vi "Camera-Events2Case.vi"(2 "OldVal":T2 {"Camera Parameters"."Pixel Format" items=["PIXEL_FORMAT_MONO8", "PIXEL_FORMAT_MONO16", "PIXEL_FORMAT_YUV422", "PIXEL_FORMAT_BAYER8_GRBG", "PIXEL_FORMAT_BAYER16_GRBG", "PIXEL_FORMAT_RGB24", "PIXEL_FORMAT_RGB48", "PIXEL_FORMAT_BAYER8_RGGB", "PIXEL_FORMAT_BAYER8_GBRG ", "PIXEL_FORMAT_BAYER8_BGGR ", "PIXEL_FORMAT_BAYER16_RGGB ", "PIXEL_FORMAT_BAYER16_GBRG", "PIXEL_FORMAT_BAYER16_BGGR", "PIXEL_FORMAT_RGB32"]}, 3 "NewVal":T2 {"Camera Parameters"."Pixel Format" items=["PIXEL_FORMAT_MONO8", "PIXEL_FORMAT_MONO16", "PIXEL_FORMAT_YUV422", "PIXEL_FORMAT_BAYER8_GRBG", "PIXEL_FORMAT_BAYER16_GRBG", "PIXEL_FORMAT_RGB24", "PIXEL_FORMAT_RGB48", "PIXEL_FORMAT_BAYER8_RGGB", "PIXEL_FORMAT_BAYER8_GBRG ", "PIXEL_FORMAT_BAYER8_BGGR ", "PIXEL_FORMAT_BAYER16_RGGB ", "PIXEL_FORMAT_BAYER16_GBRG", "PIXEL_FORMAT_BAYER16_BGGR", "PIXEL_FORMAT_RGB32"]}) -> (0 "Cameara Cambio Array":T3(array[ring]), 1 "Camara Cambio?":bool)   [LabVIEW 2010]
uses:
  <vilib>/addons/PixeLINK/Low Level Functions/CAMERA_FEATURES.llb/TDPU-CameraFeatures-PixelFormat.ctl
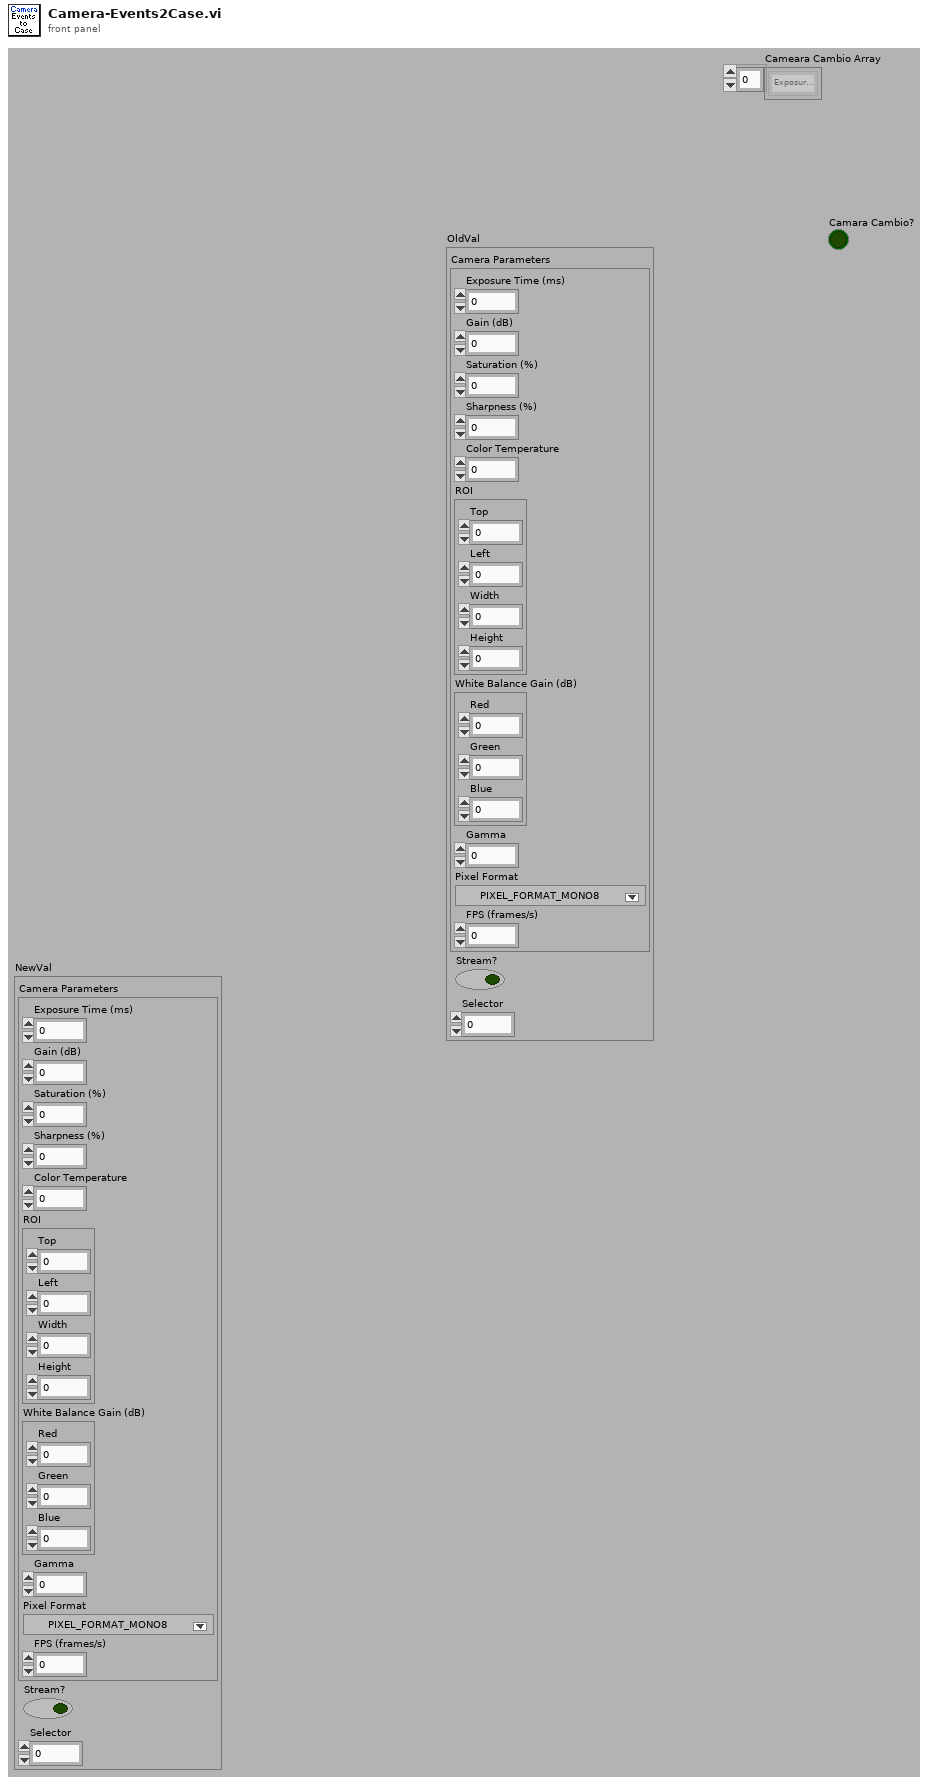
[diagram p1: front panel]
types:
  T1 = typedef "TDPU-CameraFeatures-PixelFormat.ctl" = u16
  T2 = cluster{"Camera Parameters":cluster{"Exposure Time (ms)":dbl, "Gain (dB)":dbl, "Saturation (%)":dbl, "Sharpness (%)":dbl, "Color Temperature":dbl, "ROI":cluster{"Top":i32, "Left":i32, "Width":i32, "Height":i32}, "White Balance Gain (dB)":cluster{"Red":dbl, "Green":dbl, "Blue":dbl}, "Gamma":dbl, "Pixel Format":T1, "FPS (frames/s)":i32}, "Stream?":bool, "Selector":u16}
  T3 = enum16{"Exposure Time (ms)", "Gain (dB)", "Saturation (%)", "Sharpness (%)", "Color Temperature (%)", "ROI", "White Balance Gain (dB)", "Gamma", "Pixel Format", "FPS (frames/s)", "Selector", "Stream", "Nothing"}[]
  T4 = cluster{"Top":i32, "Left":i32, "Width":i32, "Height":i32}
  T5 = enum16{"Exposure Time (ms)", "Gain (dB)", "Saturation (%)", "Sharpness (%)", "Color Temperature (%)", "ROI", "White Balance Gain (dB)", "Gamma", "Pixel Format", "FPS (frames/s)", "Selector", "Stream", "Nothing"}
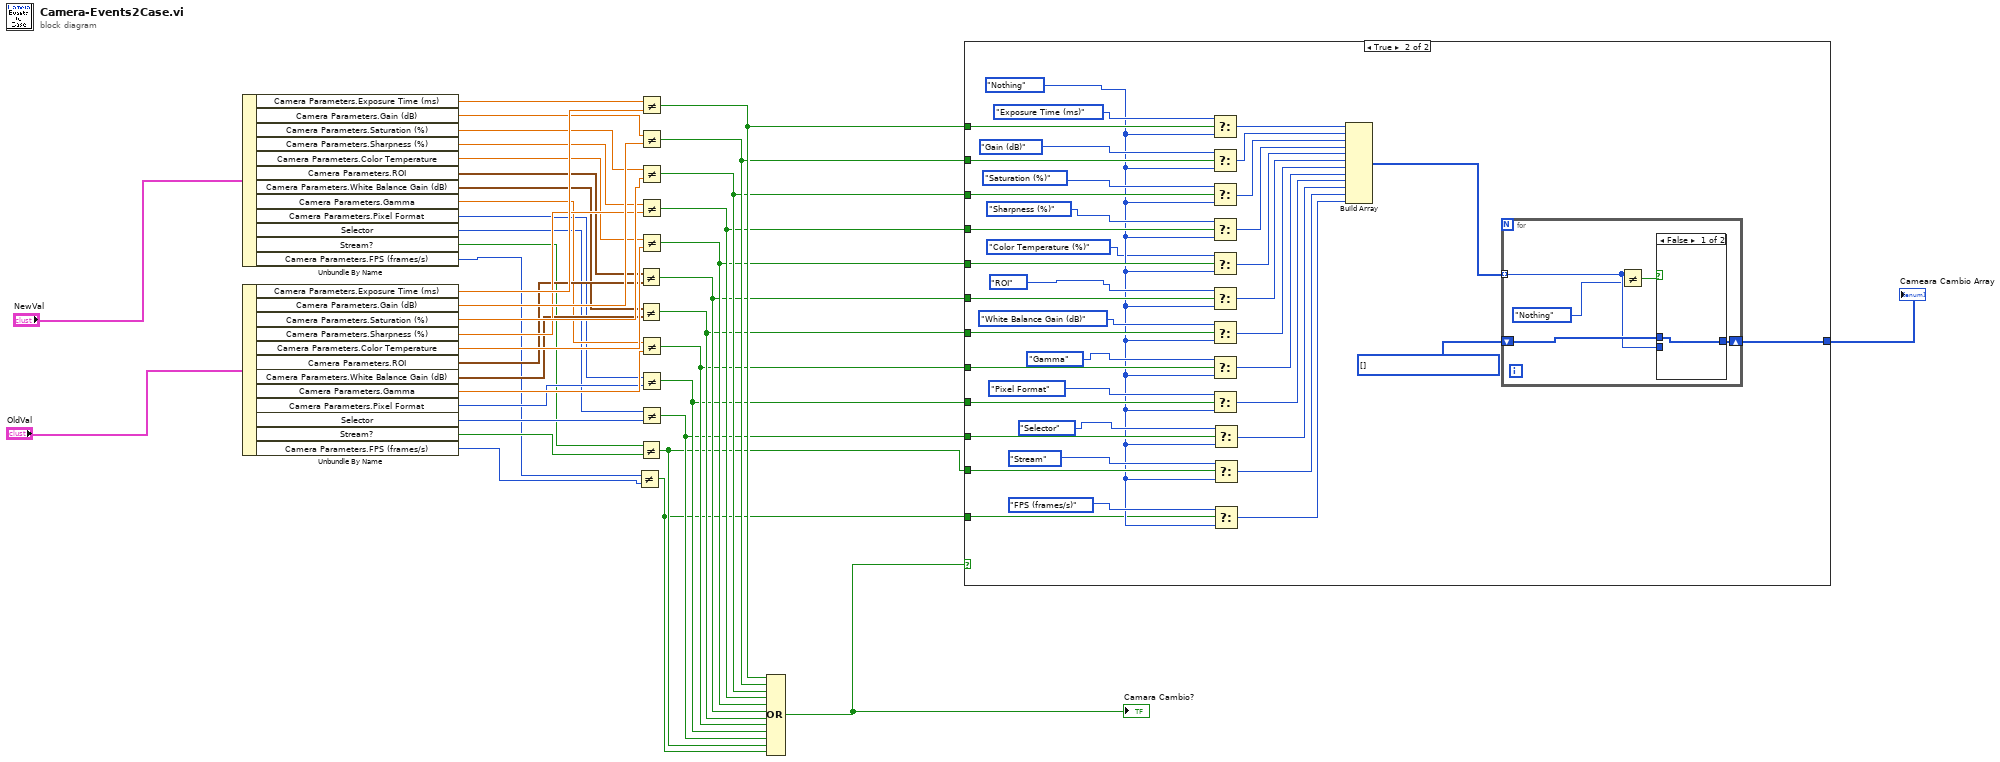
[diagram p0: block diagram]
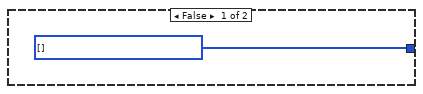
[diagram p2: hidden frame]
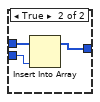
[diagram p3: hidden frame]
diagram:
  n1 = Unbundle By Name("NewVal") -> ("Camera Parameters.Exposure Time (ms)"=w40:dbl, "Camera Parameters.Gain (dB)"=w38:dbl, "Camera Parameters.Saturation (%)"=w36:dbl, "Camera Parameters.Sharpness (%)"=w34:dbl, "Camera Parameters.Color Temperature"=w32:dbl, "Camera Parameters.ROI"=w30:T4, "Camera Parameters.White Balance Gain (dB)"=w28:cluster{"Red":dbl, "Green":dbl, "Blue":dbl}, "Camera Parameters.Gamma"=w26:dbl, "Camera Parameters.Pixel Format"=w24:T1, "Selector"=w13:u16, "Stream?"=w11:bool, "Camera Parameters.FPS (frames/s)"=w5:i32)
  n2 = Unbundle By Name("OldVal") -> ("Camera Parameters.Exposure Time (ms)"=w39:dbl, "Camera Parameters.Gain (dB)"=w37:dbl, "Camera Parameters.Saturation (%)"=w35:dbl, "Camera Parameters.Sharpness (%)"=w33:dbl, "Camera Parameters.Color Temperature"=w31:dbl, "Camera Parameters.ROI"=w29:T4, "Camera Parameters.White Balance Gain (dB)"=w27:cluster{"Red":dbl, "Green":dbl, "Blue":dbl}, "Camera Parameters.Gamma"=w25:dbl, "Camera Parameters.Pixel Format"=w23:T1, "Selector"=w12:u16, "Stream?"=w10:bool, "Camera Parameters.FPS (frames/s)"=w4:i32)
  n3 = Not Equal?(x=w5, y=w4) -> (x != y?=w3:bool)
  n4 = Not Equal?(x=w30, y=w29) -> (x != y?=w17:bool)
  n5 = Not Equal?(x=w28, y=w27) -> (x != y?=w16:bool)
  n6 = Not Equal?(x=w11, y=w10) -> (x != y?=w8:bool)
  n7 = Not Equal?(x=w40, y=w39) -> (x != y?=w22:bool)
  n8 = Not Equal?(x=w38, y=w37) -> (x != y?=w21:bool)
  n9 = Not Equal?(x=w36, y=w35) -> (x != y?=w20:bool)
  n10 = Not Equal?(x=w34, y=w33) -> (x != y?=w19:bool)
  n11 = Not Equal?(x=w32, y=w31) -> (x != y?=w18:bool)
  n12 = Not Equal?(x=w26, y=w25) -> (x != y?=w15:bool)
  n13 = Not Equal?(x=w24, y=w23) -> (x != y?=w14:bool)
  n14 = Not Equal?(x=w13, y=w12) -> (x != y?=w9:bool)
  n15 = Compound Arithmetic op=OR(w22, w21, w20, w19, w18, w17, w16, w15, w14, w9, w8, w3) -> (w7:bool)
  "Camara Cambio?" <- w7
  n16 = case shown="True" w7 {
    tunnel: w22 -> [_ w71]
    tunnel: w21 -> [_ w70]
    tunnel: w20 -> [_ w69]
    tunnel: w19 -> [_ w68]
    tunnel: w18 -> [_ w67]
    tunnel: w17 -> [_ w66]
    tunnel: w16 -> [_ w65]
    tunnel: w15 -> [_ w64]
    tunnel: w14 -> [_ w63]
    tunnel: w9 -> [_ w60]
    tunnel: w8 -> [_ w59]
    tunnel: [w41 w56] -> w6
    tunnel: w3 -> [_ w43]
    frame False {
      w41 = T3 [] items=["Exposure Time (ms)", "Gain (dB)", "Saturation (%)", "Sharpness (%)", "Color Temperature (%)", "ROI", "White Balance Gain (dB)", "Gamma", "Pixel Format", "FPS (frames/s)", "Selector", "Stream", "Nothing"]
    }
    frame True {
      w45 = T5."Nothing"
      w57 = T3 [] items=["Exposure Time (ms)", "Gain (dB)", "Saturation (%)", "Sharpness (%)", "Color Temperature (%)", "ROI", "White Balance Gain (dB)", "Gamma", "Pixel Format", "FPS (frames/s)", "Selector", "Stream", "Nothing"]
      n17 = Select(t=T5."Exposure Time (ms)", s=w71, f=w45) -> (s? t:f=w80:T5)
      n18 = Select(t=T5."Gain (dB)", s=w70, f=w45) -> (s? t:f=w79:T5)
      n19 = Select(t=T5."Saturation (%)", s=w69, f=w45) -> (s? t:f=w78:T5)
      n20 = Select(t=T5."Sharpness (%)", s=w68, f=w45) -> (s? t:f=w77:T5)
      n21 = Select(t=T5."Color Temperature (%)", s=w67, f=w45) -> (s? t:f=w76:T5)
      n22 = Select(t=T5."ROI", s=w66, f=w45) -> (s? t:f=w75:T5)
      n23 = Select(t=T5."White Balance Gain (dB)", s=w65, f=w45) -> (s? t:f=w74:T5)
      n24 = Select(t=T5."Gamma", s=w64, f=w45) -> (s? t:f=w73:T5)
      n25 = Select(t=T5."Pixel Format", s=w63, f=w45) -> (s? t:f=w72:T5)
      n26 = Select(t=T5."Selector", s=w60, f=w45) -> (s? t:f=w62:T5)
      n27 = Select(t=T5."Stream", s=w59, f=w45) -> (s? t:f=w61:T5)
      n28 = Select(t=T5."FPS (frames/s)", s=w43, f=w45) -> (s? t:f=w44:T5)
      n29 = Build Array(w80, w79, w78, w77, w76, w75, w74, w73, w72, w62, w61, w44) -> (w58:T3)
      n30 = for {
        tunnel: w58 -> [w84] mode=indexing
        shift-right: [w83] -> w56
        shift-left: w57 -> [w85]
        n31 = Not Equal?(x=w84, y=T5."Nothing") -> (x != y?=w86:bool)
        n32 = case shown="False" w86 {
          tunnel: w85 -> [w87 w90]
          tunnel: w84 -> [_ w88]
          tunnel: [w87 w89] -> w83
          frame False {
          }
          frame True {
            n33 = Insert Into Array(array=w90, new element=w88) -> (w89:T3)  [unwired: 1 in]
          }
        }
      }
    }
  }
  "Cameara Cambio Array" <- w6
